vi "populate_module.vi"(11 "variable_info_in":T1) -> (3 "Module":refnum<k21>)   [LabVIEW 2015, in "Scan Engine runtime.lvclass"]
uses:
  Scan Engine runtime.lvclass
  Custom Ctrls/Index Map.ctl
  <vilib>/NI/Tag Bus/tag/Data Type.ctl
  <vilib>/NI/Tag Bus/tag/tag descriptor.lvclass
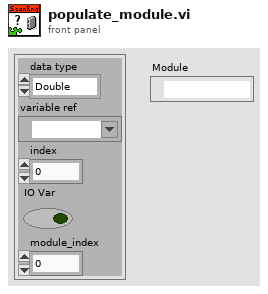
[diagram p1: front panel]
types:
  T1 = typedef "Scan Engine runtime.lvclass/Index Map.ctl" = cluster{"data type":T2, "variable ref":refnum<k21>, "index":i32, "IO Var":bool, "module_index":i32}
  T2 = typedef "tag bus.lvlib/tag descriptor.lvclass/Data Type.ctl" = enum16{"Double", "Single", "I64", "I32", "I16", "I8", "U64", "U32", "U16", "U8", "Boolean", "String", "Array of Double", "Array of Single", "Array of I64", "Array of I32", "Array of I16", "Array of I8", "Array of U64", "Array of U32", "Array of U16", "Array of U8", "Array of Boolean", "Array of String"}
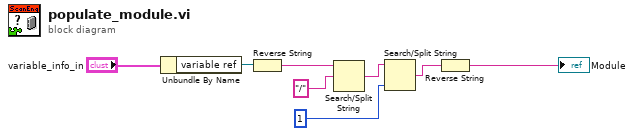
[diagram p0: block diagram]
diagram:
  n1 = Unbundle By Name("variable_info_in") -> ("variable ref"=w3:refnum<k21>)
  n2 = Reverse String(1:w3) -> (0:w7:string)
  n3 = Search/Split String(string=w7, search string/char (-)="/" ("search string")) -> (match + rest of string=w6:string)  [unwired: 1 in, 2 out]
  n4 = Search/Split String(string=w6, offset (0)=1) -> (match + rest of string=w4:string)  [unwired: 1 in, 2 out]
  n5 = Reverse String(1:w4) -> (0:→"Module":string)
